vi "Read DAQ Config Parameter.vi"(8 "error in (no error)":errorcluster, 10 "Data in":string[][][](array[string])) -> (0 "error out":errorcluster, 2 "DAQ":T1 caption="DAQ Parameter")   [LabVIEW 2016, in "DAQ IO.lvlib"]
uses:
  DAQ IO.lvlib
  DAQ Instr Config Parameter.ctl
  DI Channel Setting.ctl
  DO Channel Setting..ctl
  User Interface/User Interface.lvlib
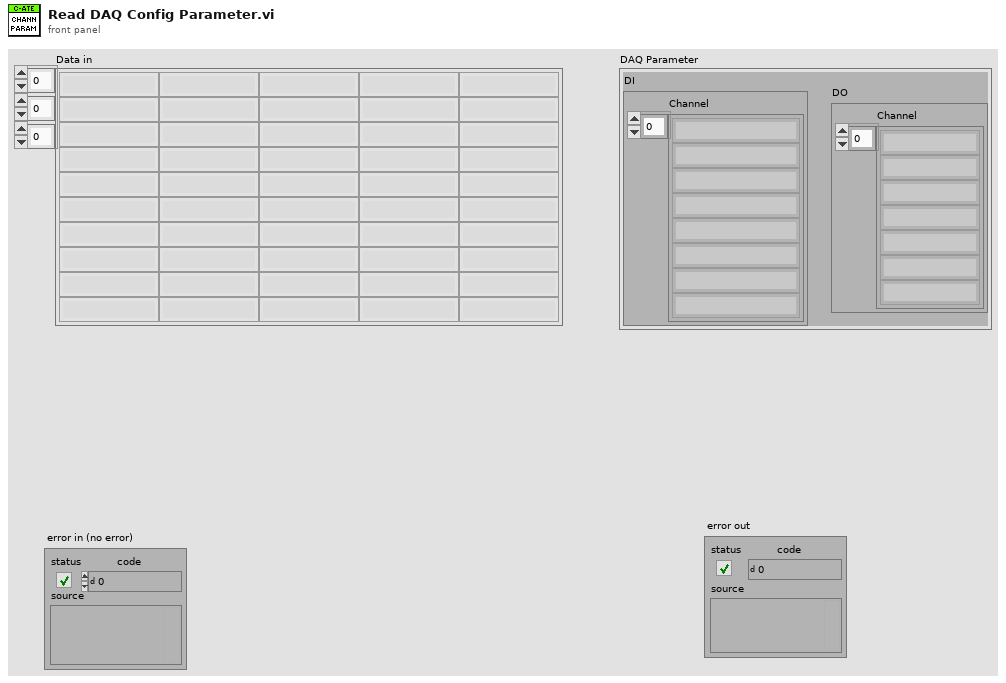
[diagram p1: front panel]
types:
  T1 = typedef "DAQ IO.lvlib/DAQ Instr Config Parameter.ctl" = cluster{"DI":T2, "DO":T3}
  T2 = typedef "DAQ IO.lvlib/DI Channel Setting.ctl" = cluster{"Channel":string[]}
  T3 = typedef "DAQ IO.lvlib/DO Channel Setting..ctl" = cluster{"Channel":string[]}
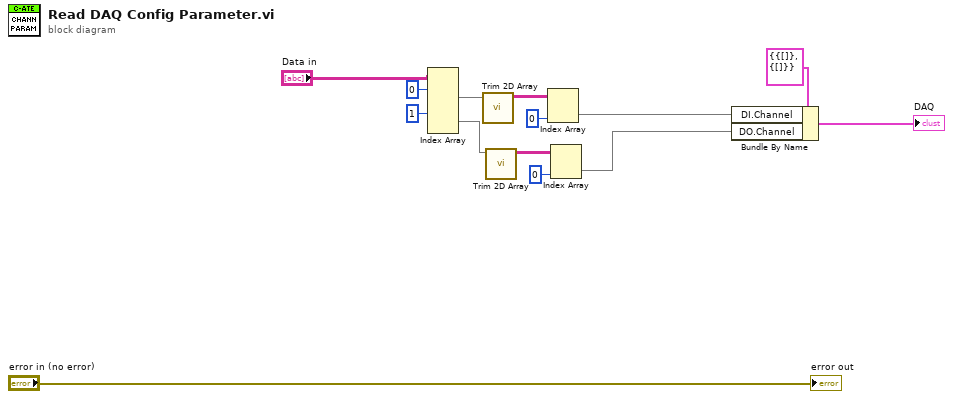
[diagram p0: block diagram]
diagram:
  n1 = Index Array(array="Data in", index (dim 0) #1=0 ("index (page)"), index (dim 0) #2=1 ("index (page)")) -> (element #1=w9:string[][], element #2=w5:string[][])  [unwired: 4 in]
  n2 = call "Trim 2D Array.vi"("Data in"=w9) -> ("Data out"=w8:string[][])  [unwired: 10 in]
  n3 = call "Trim 2D Array.vi"("Data in"=w5) -> ("Data out"=w6:string[][])  [unwired: 10 in]
  n4 = Index Array(array=w8, index (col)=0 ("disabled index (col)")) -> (element=w7:string[])  [unwired: 1 in]
  n5 = Index Array(array=w6, index (col)=0 ("disabled index (col)")) -> (element=w4:string[])  [unwired: 1 in]
  n6 = Bundle By Name(cluster=T1 {"DI"={"Channel"=[]}, "DO"={"Channel"=[]}}, "DI.Channel"=w7, "DO.Channel"=w4) -> (→"DAQ":T1)
  "error out" <- "error in (no error)"
